vi "ConcatObj.vi"(8 "error in (no error)":errorcluster, 11 "Channel in":refnum<class "Channel.lvclass">) -> (0 "error out":errorcluster, 3 "Channel out":refnum<class "Channel.lvclass">)   [LabVIEW 2018, in "Channel.lvclass"]
uses:
  Channel.lvclass
  Channel.lvclass/Channel.ctl
  Interface/Interface.lvclass
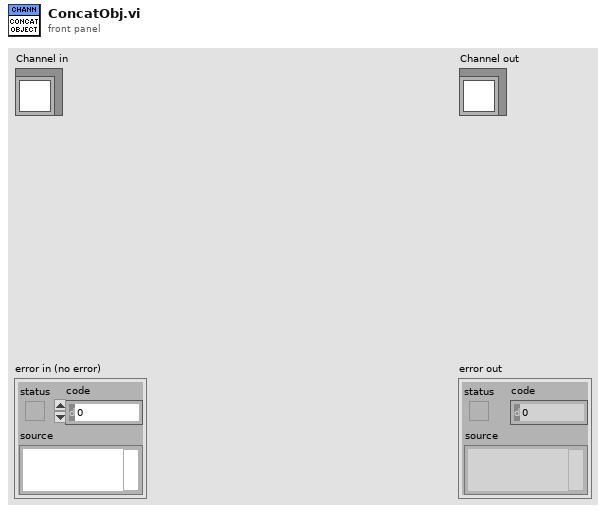
[diagram p1: front panel]
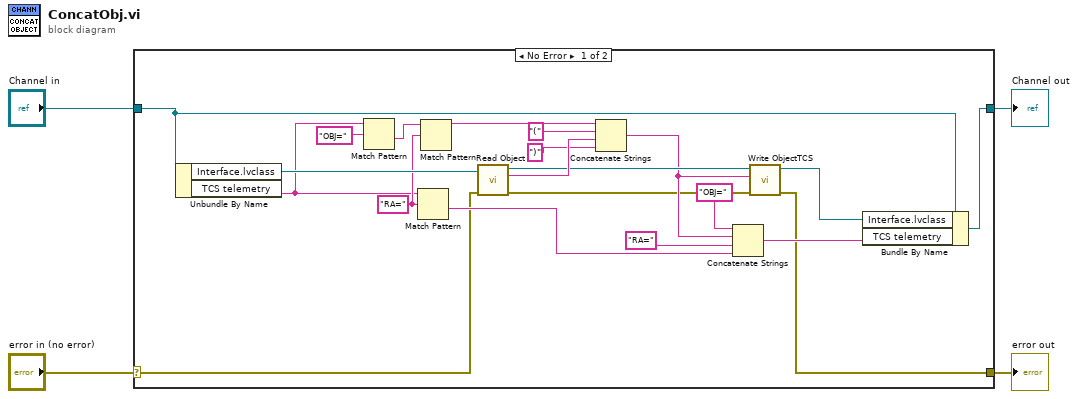
[diagram p0: block diagram]
diagram:
  n1 = case shown="No Error" "error in (no error)" {
    selector: "error in (no error)" -> [w19 w27]
    tunnel: [w5 w27] -> w3
    tunnel: [w20 w26] -> w1
    tunnel: "Channel in" -> [w22 w26]
    frame No Error {
      w18 = "RA=" ("regular expression")
      n2 = Unbundle By Name(w22) -> ("Interface.lvclass"=w25:refnum<class "Interface.lvclass">, "TCS telemetry"=w16:string)
      n3 = Match Pattern(string=w16, regular expression="OBJ=") -> (after substring=w15:string)  [unwired: 1 in, 3 out]
      n4 = Match Pattern(string=w16, regular expression=w18) -> (after substring=w23:string)  [unwired: 1 in, 3 out]
      n5 = Match Pattern(string=w15, regular expression=w18) -> (before substring=w14:string)  [unwired: 1 in, 3 out]
      n6 = call-dynamic "Read Object.vi"("error in (no error)"=w19, "Interface in"=w25) -> ("error out"=w6:errorcluster, "Object"=w12:string, "Interface out"=w9:refnum<class "Interface.lvclass">)  [unwired: 7 in]
      n7 = Concatenate Strings(w14, "(" ("string"), w12, ")" ("string")) -> (w7:string)
      n8 = Concatenate Strings("OBJ=" ("string"), w7, "RA=" ("string"), w23) -> (w21:string)
      n9 = call-dynamic "Write ObjectTCS.vi"("error in (no error)"=w6, "ObjectTCS"=w7, "Interface in"=w9) -> ("error out"=w5:errorcluster, "Interface out"=w8:refnum<class "Interface.lvclass">)  [unwired: 7 in]
      n10 = Bundle By Name(cluster=w22, "Interface.lvclass"=w8, "TCS telemetry"=w21) -> (w20:refnum<class "Channel.lvclass">)
    }
    frame Error {
    }
  }
  "error out" <- w3
  "Channel out" <- w1
